vi "Pocket UI.vi"() -> ()   [LabVIEW 2020]
uses:
  <vilib>/Utility/miscctls.llb/LVPositionTypeDef.ctl
panel:
  in  "Sliding Tab Control":enum32{"Page 2"}(tab)
  in  "Actions Button":bool
  in  "Settings Button":bool
  in  "Metrics Button":bool
  in  "Graph Button":bool
  in  "Menu Button":bool
  in  "Tab Control":T1(tab)=enum."Metrics"
  out "Waveform Graph":dynamicdata(graph)=[{"t0"=timestamp(0 s since 1904-01-01), "dt"=0.001, "Y"=[0.00170483994044508, 0.160554096670178, 0.2751956028400251, 0.08799503558302489, 0.28619937145160085, 0.5100030986392714, 0.1985780032807257, 0.3064031830706452, 0.34966550656249273, 0.35150183756271813, 0.6821879586557484, 0.5405608394777965, 0.5717511683679658, 0.5715755741452495, 0.9670340872919297, 0.8197489343472539, 0.7012738475977462, 0.8253511437824305, 0.7736745753862154, 0.80444734565485, 0.993023263767081, 1.137917880294811, 1.1069995988727492, 0.8770873718990313, 1.030924778514239, 1.0634343352593396, 0.8401334855133229, 1.1518028732628398, 0.9700200409987094, 0.8026807491784901, 0.8183695588828049, 0.9520465738081972, 0.857783346508061, 0.9688916960873557, 0.7670146474609557, 0.9401001653861989, 0.7180783877295495, 0.8560519170415788, 0.701921130546114, 0.7208145308157821, 0.6110139610407335, 0.32979217269692795, 0.5099592439812186, 0.3902024868474646, 0.5322392085175534, 0.2612497195186862, 0.32874372233372795, 0.20390061585668987, 0.18214219196360665, 0.07441413538163949, 0.16822594383801337, -0.19626396737964216, -0.2082188568290131, -0.22149872566782297, -0.4699802990333111, -0.43848419395538446, -0.5651982606844008, -0.6189523280180936, -0.5750858662243751, -0.5517097051444678, -0.4641167386062769, -0.6432077868410019, -0.7480717925640029, -0.8460291823844561, -0.7097021596210032, -0.6609919532893181, -1.0648009409056285, -0.9213562855867193, -0.8065524924012425, -1.0247855737007932, -1.0246888456767744, -0.8781171564356188, -0.9706167884167879, -0.8643357340938744, -1.059532850901939, -0.8567992636147913, -0.8666507842216239, -0.7944351423123155, -1.1643103747904342, -1.1227750789930608, -0.8377190002662311, -1.0305550874886933, -0.7621214646664622, -1.0388953896150523, -0.809330681199577, -0.922816835416193, -0.7502153457679688, -0.7332555280869756, -0.7952271228819697, -0.5407018854773732, -0.6892513539851433, -0.5369769293551574, -0.6090071571818626, -0.1971441902377854, -0.23352012566618618, -0.3188572433888205, -0.2876729332679234, -0.032711455572667664, 0.1207437458666783, -0.19310420981005838], "attributes"=variant("NI_ChannelName"=variant(string "Sine with Uniform Noise"), "NI_ExpIsRelativeTime"=variant(bool TRUE), "NI_ExpStartTimeStamp"=variant(timestamp timestamp(3347901195.5745254 s since 1904-01-01)), "NI_ExpTimeStamp"=variant(timestamp timestamp(3347901195.5745254 s since 1904-01-01)), "NI_ExpXDimension"=variant(string "t"))}]
  out "Life, the Universe,\nand Everything":dbl=42.0
  in  "stop":bool
  in  "Numeric":dbl
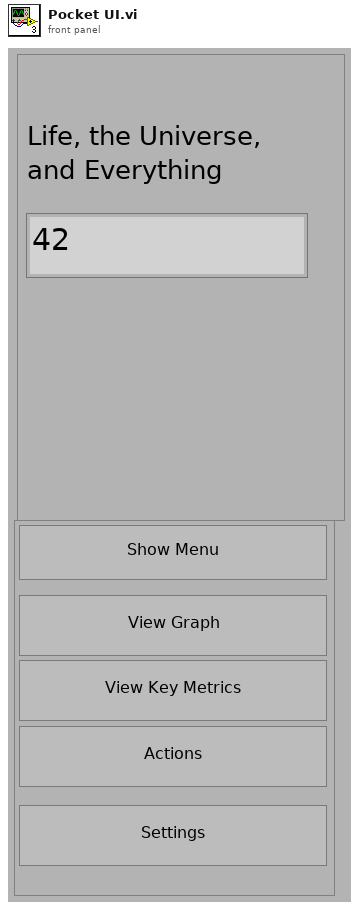
[diagram p1: front panel]
types:
  T1 = enum32{"Graph", "Metrics", "Actions", "Settings"}
  T2 = typedef "LVPositionTypeDef.ctl" = cluster{"Left":i32, "Top":i32}
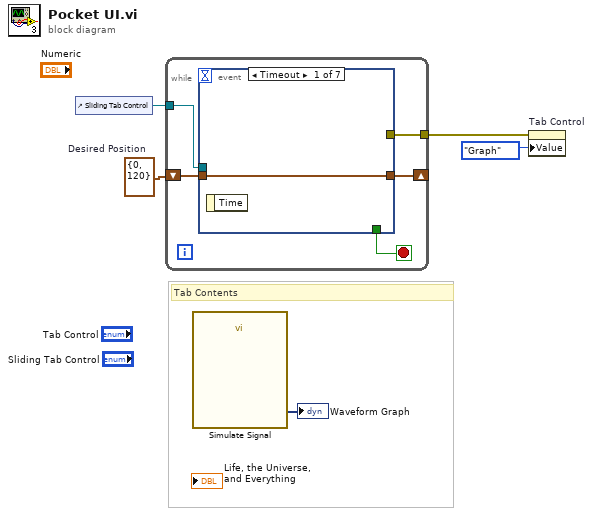
[diagram p0: block diagram]
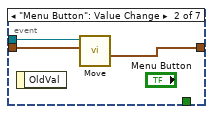
[diagram p2: hidden frame]
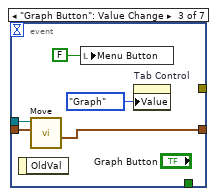
[diagram p3: hidden frame]
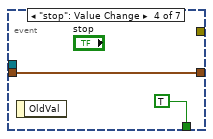
[diagram p4: hidden frame]
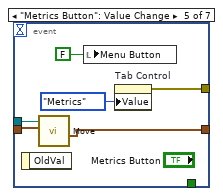
[diagram p5: hidden frame]
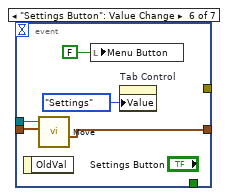
[diagram p6: hidden frame]
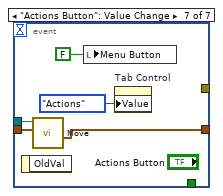
[diagram p7: hidden frame]
diagram:
  w5 = T2 {"Left"=0, "Top"=120}  # Desired Position
  # "Tab Contents"
  n1 = control-ref of="Sliding Tab Control"() -> (w4:refnum<vi>)
  n2 = while {
    shift-right: [w8] -> _
    shift-left: w5 -> [w10]
    tunnel: w4 -> [w9]
    tunnel: [w6] -> w2
    stop <- w7 stop-if-true
    n3 = event shown="[0] Timeout" {
      selector: _ -> [_ _ _ _ _ _ _]
      dyn-events: _ -> [_ _ _ _ _ _ _]
      timeout: _ -> [_ _ _ _ _ _ _]
      tunnel: w10 -> [w11 w14 w18 w21 w25 w30 w35]
      tunnel: w9 -> [_ w13 w16 _ w26 w31 w36]
      tunnel: [w11 w12 w17 w21 w24 w29 w34] -> w8
      tunnel: [_ _ _ TRUE _ _ _] -> w7
      tunnel: [_ _ _ _ w22 _ _] -> w6
      event Timeout {
        n4 = event-data() -> ()  [unwired: 1 in, 1 out]
      }
      event "Menu Button": Value Change {
        n5 = event-data() -> ()  [unwired: 1 in, 1 out]
        n6 = call "Move.vi"("Desired Position"=w14, "Obj Ref"=w13) -> ("Old Position"=w12:T2)  [unwired: 7 in, 2 out]
      }
      event "Graph Button": Value Change {
        n7 = event-data() -> ()  [unwired: 1 in, 1 out]
        n8 = call "Move.vi"("Desired Position"=w18, "Obj Ref"=w16) -> ("Old Position"=w17:T2)  [unwired: 7 in, 2 out]
        n9 = local write "Menu Button"(FALSE ("Menu Button")) -> ()
        n10 = property on="Tab Control" class="TabCtl (strict)"("Value"=T1."Graph" ("Tab Control")) -> ()  [unwired: 2 in, 2 out]
      }
      event "stop": Value Change {
        n11 = event-data() -> ()  [unwired: 1 in, 1 out]
      }
      event "Metrics Button": Value Change {
        n12 = event-data() -> ()  [unwired: 1 in, 1 out]
        n13 = call "Move.vi"("Desired Position"=w25, "Obj Ref"=w26) -> ("Old Position"=w24:T2)  [unwired: 7 in, 2 out]
        n14 = local write "Menu Button"(FALSE ("Menu Button")) -> ()
        n15 = property on="Tab Control" class="TabCtl (strict)"("Value"=T1."Metrics" ("Tab Control")) -> (error out=w22:errorcluster)  [unwired: 2 in, 1 out]
      }
      event "Settings Button": Value Change {
        n16 = event-data() -> ()  [unwired: 1 in, 1 out]
        n17 = call "Move.vi"("Desired Position"=w30, "Obj Ref"=w31) -> ("Old Position"=w29:T2)  [unwired: 7 in, 2 out]
        n18 = local write "Menu Button"(FALSE ("Menu Button")) -> ()
        n19 = property on="Tab Control" class="TabCtl (strict)"("Value"=T1."Settings" ("Tab Control")) -> ()  [unwired: 2 in, 2 out]
      }
      event "Actions Button": Value Change {
        n20 = event-data() -> ()  [unwired: 1 in, 1 out]
        n21 = call "Move.vi"("Desired Position"=w35, "Obj Ref"=w36) -> ("Old Position"=w34:T2)  [unwired: 7 in, 2 out]
        n22 = local write "Menu Button"(FALSE ("Menu Button")) -> ()
        n23 = property on="Tab Control" class="TabCtl (strict)"("Value"=T1."Actions" ("Tab Control")) -> ()  [unwired: 2 in, 2 out]
      }
    }
  }
  n24 = call "Simulate Signal"() -> ("Sine with Uniform Noise"=→"Waveform Graph":dynamicdata)  [unwired: 14 in, 1 out]
  n25 = property on="Tab Control" class="TabCtl (strict)"(error in=w2, "Value"=T1."Graph" ("Tab Control")) -> ()  [unwired: 1 in, 2 out]
